vi "IdentifyAndReadInstr.vi"(8 "error in (no error)":errorcluster, 11 "VISA Resource Name":refnum<visa-resource-name>) -> (0 "error out":errorcluster, 1 "Instrument":T1=enum."LkShr 340 chA&B", 2 "Identified":bool, 3 "VISA Resource Name Out":refnum<visa-resource-name>)   [LabVIEW 2018]
uses:
  Device/Device type.ctl
  GPIB/VISA  Send Receive.vi
  <vilib>/Utility/error.llb/Error Cluster From Error Code.vi
  <vilib>/ErrorRing/Error Ring.xnode
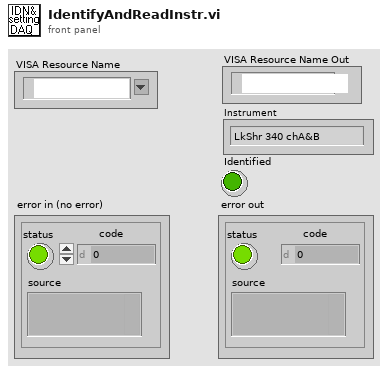
[diagram p1: front panel]
types:
  T1 = typedef "Device type.ctl" = enum16{"NONE", "Neocera 21", "LakeShore 335", "LakeShore 336", "LakeShore 340", "LkShr 340 chA&B", "LakeShore 370", "SRS 850", "SRS 830", "LR 700", "EG&G 5302", "EG&G 7260", "EG&G 7280", "AH 2500", "AH 2550", "AH 2700", "Keithley meter", "Keithley electrometer", "Keithley 182", "HP 5385", "HP 53181", "HP 53132", "ITC503", "IPS120", "Oxford Mercury IPS", "Oxford PS", "Test", "DC Facility Magnet", "Cryomagnetics PS", "Keithley 2400", "Keithley current source", "Cryo-Con 22C", "HP87NN", "HP4395A", "Agilent 34410A", "Arduino TC"}
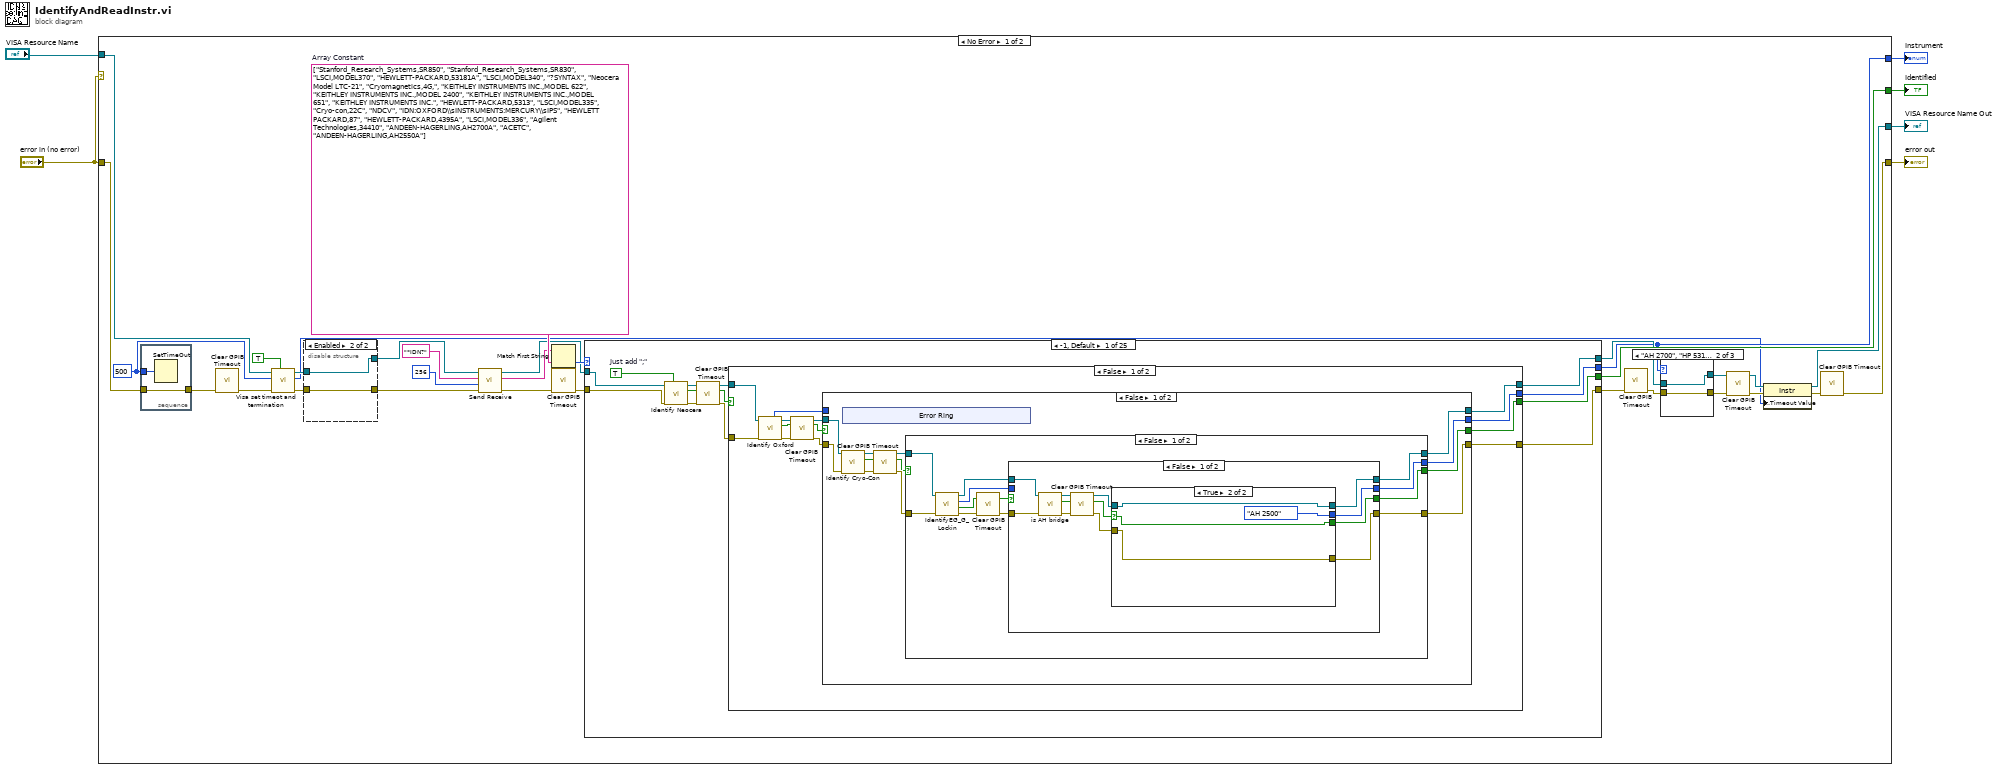
[diagram p0: block diagram]
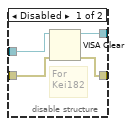
[diagram p2: hidden frame]
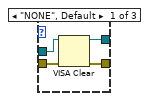
[diagram p3: hidden frame]
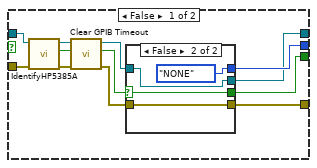
[diagram p5: hidden frame]
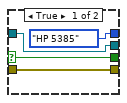
[diagram p6: hidden frame]
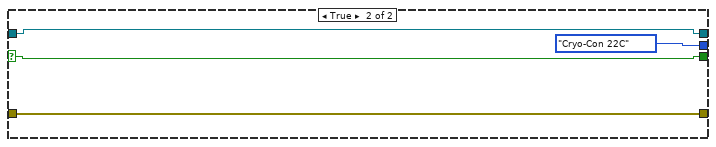
[diagram p8: hidden frame]
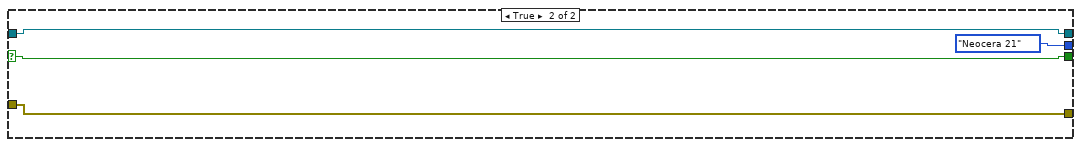
[diagram p10: hidden frame]
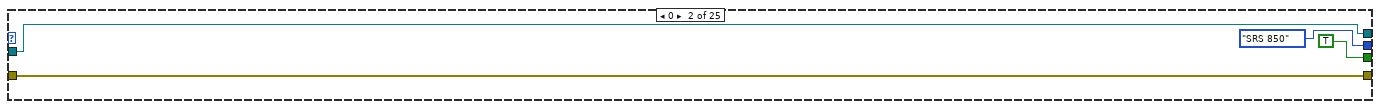
[diagram p11: hidden frame]
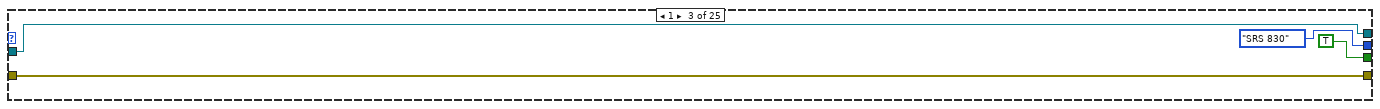
[diagram p12: hidden frame]
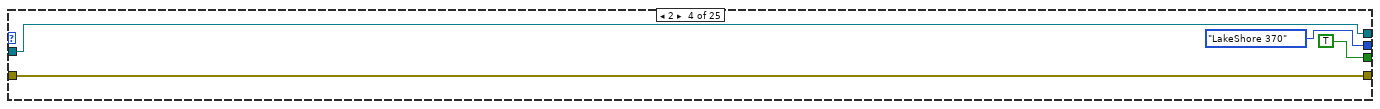
[diagram p13: hidden frame]
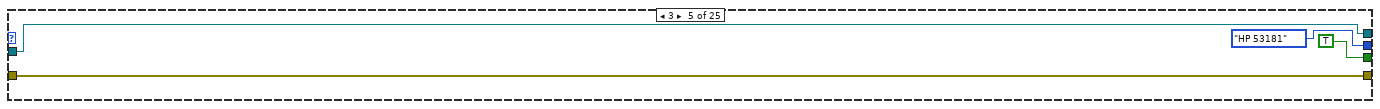
[diagram p14: hidden frame]
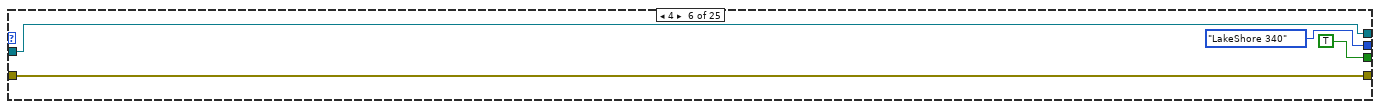
[diagram p15: hidden frame]
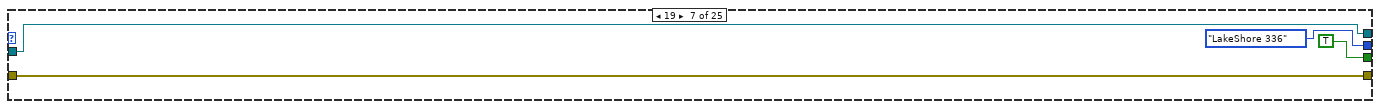
[diagram p16: hidden frame]
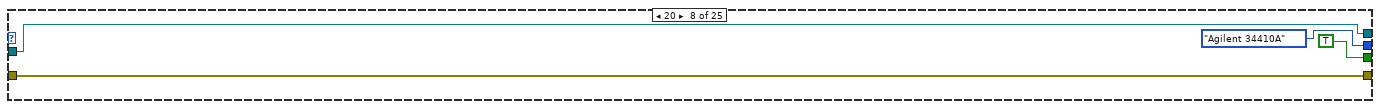
[diagram p17: hidden frame]
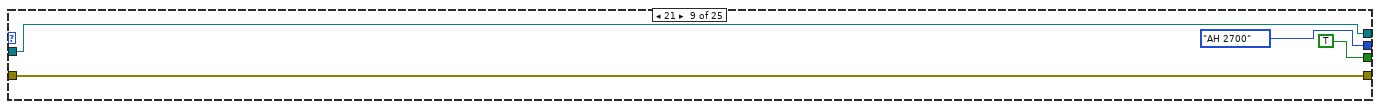
[diagram p18: hidden frame]
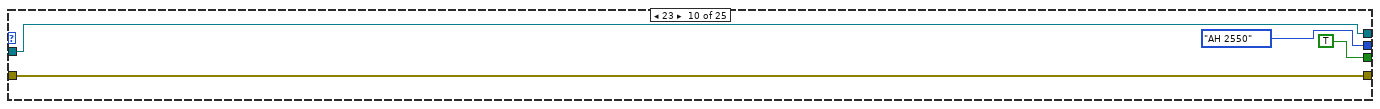
[diagram p19: hidden frame]
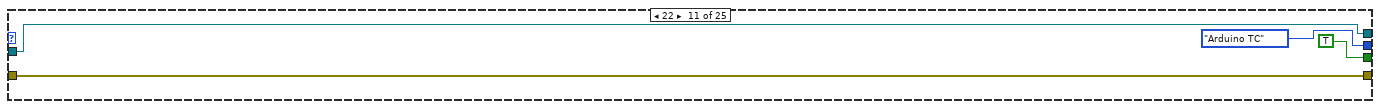
[diagram p20: hidden frame]
diagram:
  n1 = case shown="No Error" "error in (no error)" {
    tunnel: "error in (no error)" -> [w28 w259]
    tunnel: [w15 w259] -> w3
    tunnel: [w31 FALSE ("Identified")] -> w6
    tunnel: [w21 Device_type."NONE" ("Instrument")] -> w1
    tunnel: "VISA Resource Name" -> [w13 w257]
    tunnel: [w14 w257] -> w2
    frame No Error {
      w36 = string[] ["Stanford_Research_Systems,SR850", "Stanford_Research_Systems,SR830", "LSCI,MODEL370", "HEWLETT-PACKARD,53181A", "LSCI,MODEL340", "?SYNTAX", "Neocera Model LTC-21", "Cryomagnetics,4G,", "KEITHLEY INSTRUMENTS INC.,MODEL 622", "KEITHLEY INSTRUMENTS INC.,MODEL 2400", "KEITHLEY INSTRUMENTS INC.,MODEL 651", "KEITHLEY INSTRUMENTS INC.", "HEWLETT-PACKARD,5313", "LSCI,MODEL335", "Cryo-con,22C", "NDCV", "IDN:OXFORD\\sINSTRUMENTS:MERCURY\\sIPS", "HEWLETT PACKARD,87", "HEWLETT-PACKARD,4395A", "LSCI,MODEL336", "Agilent Technologies,34410", "ANDEEN-HAGERLING,AH2700A", "ACETC", "ANDEEN-HAGERLING,AH2550A"]  # Array Constant
      w7 = 500 ("new timeout (10000)")
      n2 = stacked-sequence {
        tunnel: w28 -> [w52]
        tunnel: [w52] -> w16
        tunnel: w7 -> [w51]
        frame #0 {
          n3 = SetTimeOut(1:w51) -> ()  [unwired: 1 out]
        }
      }
      n4 = call "Clear GPIB Timeout.vi"("error in (no error)"=w16) -> ("error out"=w9:errorcluster)  [unwired: 1 in, 9 out]
      n5 = call "Visa set timeot and termination.vi"("Termination Character Enable Based on Interface"=TRUE, "error in (no error)"=w9, "Timeout Value"=w7, "VISA resource name"=w13) -> ("error out"=w8:errorcluster, "Old Timeout Value"=w11:u32, "VISA resource name out"=w12:refnum<visa-resource-name>)  [unwired: 3 in, 2 out]
      n6 = disable-structure shown="Enabled" {
        disable-tunnel: w8 -> [w40 w41]
        disable-tunnel: w12 -> [w39 w42]
        disable-tunnel: [w38 w42] -> w18
        disable-tunnel: [w37 w41] -> w17
        frame Disabled {
          # "For\nKei182"
          n7 = VISA Clear(VISA resource name=w39, error in (no error)=w40) -> (VISA resource name out=w38:refnum<visa-resource-name>, error out=w37:errorcluster)
        }
        frame Enabled {
        }
      }
      n8 = call-poly "Send Receive.vi"("error in (no error)"=w17, "Receive count"=256 ("count"), "data string in"="*IDN?" ("data string"), "VISA Resource Name"=w18) -> ("error out"=w33:errorcluster, "data string out"=w32:string, "VISA Resource Name Out"=w27:refnum<visa-resource-name>)  [unwired: 5 in]
      n9 = Match First String(2:w36, 3:w32) -> (0:w35:i32)  [unwired: 1 out]
      n10 = call "Clear GPIB Timeout.vi"("error in (no error)"=w33) -> ("error out"=w30:errorcluster)  [unwired: 1 in, 9 out]
      n11 = case shown="-1, Default" w35 {
        tunnel: w30 -> [w59 w150 w154 w158 w162 w166 w170 w174 w178 w182 w186 w190 w194 w198 w202 w206 w212 w217 w221 w225 w229 w232 w244 w248 w252]
        tunnel: [w63 w150 w154 w158 w162 w166 w170 w174 w178 w182 w186 w190 w194 w198 w202 w206 w209 w217 w221 w225 w229 w231 w244 w248 w252] -> w26
        tunnel: [w61 TRUE ("Identified") TRUE ("Identified") TRUE ("Identified") TRUE ("Identified") TRUE ("Identified") TRUE ("Identified") TRUE ("Identified") TRUE ("Identified") TRUE ("Identified") TRUE ("Identified") TRUE ("Identified") TRUE ("Identified") TRUE ("Identified") TRUE ("Identified") TRUE ("Identified") TRUE ("Identified") TRUE ("Identified") TRUE ("Identified") TRUE ("Identified") TRUE ("Identified") TRUE ("Identified") TRUE ("Identified") TRUE ("Identified") TRUE ("Identified")] -> w31
        tunnel: [w62 Device_type."SRS 850" ("Instrument") Device_type."SRS 830" ("Instrument") Device_type."LakeShore 370" ("Instrument") Device_type."HP 53181" ("Instrument") Device_type."LakeShore 340" ("Instrument") Device_type."LakeShore 336" ("Instrument") Device_type."Agilent 34410A" ("Instrument") Device_type."AH 2700" ("Instrument") Device_type."AH 2550" ("Instrument") Device_type."Arduino TC" ("Instrument") Device_type."LR 700" ("Instrument") Device_type."Neocera 21" ("Instrument") Device_type."Cryomagnetics PS" ("Instrument") Device_type."Keithley current source" ("Instrument") Device_type."Keithley 2400" ("Instrument") Device_type."Keithley electrometer" ("Instrument") Device_type."Keithley meter" ("Instrument") Device_type."HP 53132" ("Instrument") Device_type."LakeShore 335" ("Instrument") Device_type."Cryo-Con 22C" ("Instrument") Device_type."Keithley 182" ("Instrument") Device_type."Oxford Mercury IPS" ("Instrument") Device_type."HP87NN" ("Instrument") Device_type."HP4395A" ("Instrument")] -> w21
        tunnel: w27 -> [w56 w149 w153 w157 w161 w165 w169 w173 w177 w181 w185 w189 w193 w197 w201 w205 w211 w216 w220 w224 w228 w235 w245 w249 w253]
        tunnel: [w60 w149 w153 w157 w161 w165 w169 w173 w177 w181 w185 w189 w193 w197 w201 w205 w208 w216 w220 w224 w228 w233 w245 w249 w253] -> w24
        frame -1, Default {
          w53 = TRUE  # Just add ";"
          n12 = call "Identify Neocera.vi"("Just add \";\""=w53, "error in (no error)"=w59, "VISA Resource Name"=w56) -> ("error out"=w58:errorcluster, "Identified"=w54:bool, "VISA Resource Name Out"=w55:refnum<visa-resource-name>)  [unwired: 5 in, 1 out]
          n13 = call "Clear GPIB Timeout.vi"("error in (no error)"=w58) -> ("error out"=w57:errorcluster)  [unwired: 1 in, 9 out]
          n14 = case shown="False" w54 {
            selector: w54 -> [_ w144]
            tunnel: [w74 w145] -> w63
            tunnel: w57 -> [w64 w145]
            tunnel: [w73 Device_type."Neocera 21" ("Instrument")] -> w62
            tunnel: [w72 w144] -> w61
            tunnel: [w71 w146] -> w60
            tunnel: w55 -> [w70 w146]
            frame False {
              n15 = call "Identify Oxford.vi"("Error In"=w64, "VISA resource name"=w70) -> ("Error Out"=w68:errorcluster, "It's from Oxford!"=w66:bool, "VISA resource name out"=w69:refnum<visa-resource-name>, "Instrument"=w65:T1)  [unwired: 5 in, 1 out]
              n16 = call "Clear GPIB Timeout.vi"("error in (no error)"=w68) -> ("error out"=w67:errorcluster)  [unwired: 1 in, 9 out]
              n17 = case shown="False" w66 {
                selector: w66 -> [_ w142]
                tunnel: [w84 w143] -> w74
                tunnel: [w83 w140] -> w73
                tunnel: [w82 w142] -> w72
                tunnel: [w81 w141] -> w71
                tunnel: w69 -> [w77 w141]
                tunnel: w67 -> [w79 w143]
                tunnel: w65 -> [_ w140]
                frame False {
                  n18 = call "Identify Cryo-Con.vi"("Error In"=w79, "VISA resource name"=w77) -> ("Error Out"=w78:errorcluster, "Cryo-con"=w75:bool, "VISA resource name out"=w76:refnum<visa-resource-name>)  [unwired: 6 in, 1 out]
                  n19 = xnode "Error Ring"() -> ()  [unwired: 1 out]
                  n20 = call "Clear GPIB Timeout.vi"("error in (no error)"=w78) -> ("error out"=w80:errorcluster)  [unwired: 1 in, 9 out]
                  n21 = case shown="False" w75 {
                    selector: w75 -> [_ w137]
                    tunnel: [w99 w138] -> w84
                    tunnel: w80 -> [w98 w138]
                    tunnel: [w96 Device_type."Cryo-Con 22C" ("Instrument")] -> w83
                    tunnel: [w95 w137] -> w82
                    tunnel: w76 -> [w91 w139]
                    tunnel: [w89 w139] -> w81
                    frame False {
                      n22 = call "IdentifyEG_G_Lockin.vi"("error in (no error)"=w98, "VISA Resource Name"=w91) -> ("error out"=w97:errorcluster, "Identified"=w92:bool, "Instrument"=w94:T1, "VISA Resource Name Out"=w90:refnum<visa-resource-name>)  [unwired: 6 out]
                      n23 = call "Clear GPIB Timeout.vi"("error in (no error)"=w97) -> ("error out"=w93:errorcluster)  [unwired: 1 in, 9 out]
                      n24 = case shown="False" w92 {
                        selector: w92 -> [_ w132]
                        tunnel: [w105 w135] -> w99
                        tunnel: w93 -> [w109 w135]
                        tunnel: [w103 w134] -> w96
                        tunnel: [w108 w132] -> w95
                        tunnel: w94 -> [_ w134]
                        tunnel: w90 -> [w102 w133]
                        tunnel: [w100 w133] -> w89
                        frame False {
                          n25 = call "is AH bridge.vi"("Error In"=w109, "VISA resource name"=w102) -> ("Error Out"=w106:errorcluster, "Is AH?"=w107:bool, "VISA resource name out"=w101:refnum<visa-resource-name>)  [unwired: 7 out]
                          n26 = call "Clear GPIB Timeout.vi"("error in (no error)"=w106) -> ("error out"=w104:errorcluster)  [unwired: 1 in, 9 out]
                          n27 = case shown="True" w107 {
                            selector: w107 -> [_ w128]
                            tunnel: [w118 Device_type."AH 2500" ("Instrument")] -> w103
                            tunnel: [w110 w128] -> w108
                            tunnel: w104 -> [w119 w131]
                            tunnel: [w112 w131] -> w105
                            tunnel: w101 -> [w117 w130]
                            tunnel: [w111 w130] -> w100
                            frame False {
                              n28 = call "IdentifyHP5385A.vi"("error in (no error)"=w119, "VISA Resource Name"=w117) -> ("error out"=w114:errorcluster, "Identified"=w116:bool, "VISA Resource Name Out"=w115:refnum<visa-resource-name>)  [unwired: 7 out]
                              n29 = call "Clear GPIB Timeout.vi"("error in (no error)"=w114) -> ("error out"=w113:errorcluster)  [unwired: 1 in, 9 out]
                              n30 = case shown="False" w116 {
                                selector: w116 -> [w120 w124]
                                tunnel: [Device_type."HP 5385" ("Instrument") Device_type."NONE" ("Instrument")] -> w118
                                tunnel: w113 -> [w121 w125]
                                tunnel: w115 -> [w122 w126]
                                tunnel: [w121 w125] -> w112
                                tunnel: [w122 w126] -> w111
                                tunnel: [w120 w124] -> w110
                                frame True {
                                }
                                frame False {
                                }
                              }
                            }
                            frame True {
                            }
                          }
                        }
                        frame True {
                        }
                      }
                    }
                    frame True {
                    }
                  }
                }
                frame True {
                }
              }
            }
            frame True {
            }
          }
        }
        frame 0 {
        }
        frame 1 {
        }
        frame 2 {
        }
        frame 3 {
        }
        frame 4 {
        }
        frame 19 {
        }
        frame 20 {
        }
        frame 21 {
        }
        frame 23 {
        }
        frame 22 {
        }
        frame 5 {
        }
        frame 6 {
        }
        frame 7 {
        }
        frame 8 {
        }
        frame 9 {
        }
        frame 10 {
          n31 = VISA Write(VISA resource name=w211, write buffer=":INIT", error in (no error)=w212) -> (VISA resource name out=w208:refnum<visa-resource-name>, error out=w209:errorcluster)  [unwired: 1 out]
        }
        frame 11 {
        }
        frame 12 {
        }
        frame 13 {
        }
        frame 14 {
        }
        frame 15 {
          n32 = disable-structure shown="Disabled" {
            disable-tunnel: w235 -> [w241 w243]
            disable-tunnel: [w240 w243] -> w233
            disable-tunnel: w232 -> [w239 w242]
            disable-tunnel: [w238 w242] -> w231
            frame Disabled {
              # "Skip prefix in returnet data"
              n33 = VISA Write(VISA resource name=w241, write buffer="G0", error in (no error)=w239) -> (VISA resource name out=w240:refnum<visa-resource-name>, error out=w238:errorcluster)  [unwired: 1 out]
            }
            frame Enabled {
            }
          }
        }
        frame 16 {
        }
        frame 17 {
        }
        frame 18 {
        }
      }
      n34 = call "Clear GPIB Timeout.vi"("error in (no error)"=w26) -> ("error out"=w25:errorcluster)  [unwired: 1 in, 9 out]
      n35 = case shown="\"AH 2700\", \"HP 53181\", \"HP 53132\"" w21 {
        tunnel: w25 -> [w46 w48 w50]
        tunnel: w24 -> [w45 w47 w49]
        tunnel: [w44 w48 w50] -> w20
        tunnel: [w43 w47 w49] -> w22
        frame "NONE", Default {
          n36 = VISA Clear(VISA resource name=w45, error in (no error)=w46) -> (VISA resource name out=w43:refnum<visa-resource-name>, error out=w44:errorcluster)
        }
        frame "AH 2700", "HP 53181", "HP 53132" {
        }
        frame "Keithley meter" {
        }
      }
      n37 = call "Clear GPIB Timeout.vi"("error in (no error)"=w20) -> ("error out"=w19:errorcluster)  [unwired: 1 in, 9 out]
      n38 = property class="Instr"(reference=w22, error in=w19, "General Settings:Timeout Value"=w11) -> (reference out=w14:refnum<visa-resource-name>, error out=w23:errorcluster)
      n39 = call "Clear GPIB Timeout.vi"("error in (no error)"=w23) -> ("error out"=w15:errorcluster)  [unwired: 8 in, 2 out]
    }
    frame Error {
    }
  }
  "error out" <- w3
  "Identified" <- w6
  "Instrument" <- w1
  "VISA Resource Name Out" <- w2
